vi "Meas.vi"(8 "error in (no error)":errorcluster, 10 "Variable":enum16{"Voltage", "Current"}(ring), 11 "Connection in":T1={"Baud"=9600, "Flow Ctl"=0, "COM port"="", "Parity"=0} {"Parity" items=["None", "Odd", "Even"]; "Flow Ctl" items=["None"]; "Baud" items=["4800"=4800, "9600"=9600, "19200"=19200, "38400"=38400]}) -> (0 "error out":errorcluster, 2 "Value":dbl, 3 "Connection out":T1={"Baud"=9600, "Flow Ctl"=0, "COM port"="", "Parity"=0} {"Parity" items=["None", "Odd", "Even"]; "Flow Ctl" items=["None"]; "Baud" items=["4800"=4800, "9600"=9600, "19200"=19200, "38400"=38400]})   [LabVIEW 2014, in "B&K Precision 9120 series.lvclass"]
uses:
  B&K Precision 9120 series.lvclass
  Serial_Config.ctl
  <vilib>/Utility/error.llb/DialogType.ctl
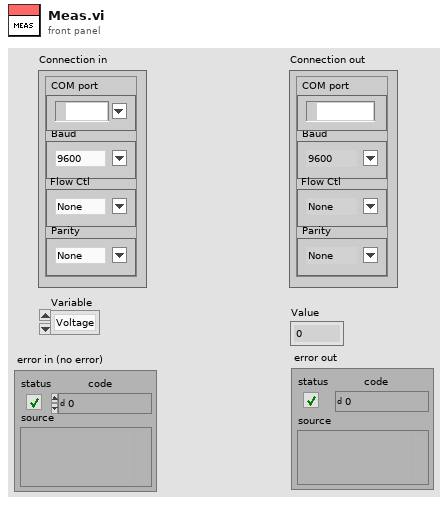
[diagram p1: front panel]
types:
  T1 = typedef "B&K Precision 9120 series.lvclass/Serial_Config.ctl" = cluster{"Baud":u32, "Flow Ctl":u16, "COM port":refnum<visa-resource-name>, "Parity":u16}
  T2 = typedef "DialogType.ctl" = u16
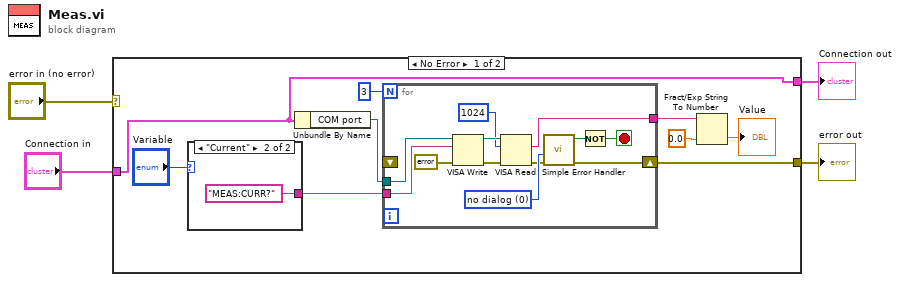
[diagram p0: block diagram]
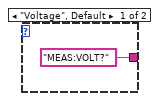
[diagram p2: hidden frame]
diagram:
  n1 = case shown="No Error" "error in (no error)" {
    selector: "error in (no error)" -> [_ w29]
    tunnel: [w6 w29] -> w4
    tunnel: "Connection in" -> [w5 w28]
    tunnel: [w5 w28] -> w1
    frame No Error {
      n2 = case shown="\"Current\"" "Variable" {
        tunnel: ["MEAS:VOLT?" ("write buffer") "MEAS:CURR?" ("write buffer")] -> w13
        frame "Voltage", Default {
        }
        frame "Current" {
        }
      }
      n3 = Unbundle By Name(w5) -> ("COM port"=w9:refnum<visa-resource-name>)
      n4 = for {
        N: 3 -> [_]
        tunnel: w13 -> [w24]
        tunnel: [w22] -> w11
        tunnel: w9 -> [w21]
        shift-right: [w15] -> w6
        shift-left: _ -> [_]
        stop <- w16 stop-if-true
        w19 = T2 0 items=["no dialog", "OK message", "continue or stop message", "OK message + warnings", "continue/stop + warnings"] ("type of dialog (OK msg:1)")
        n5 = VISA Write(VISA resource name=w21, write buffer=w24, error in (no error)=errorcluster {"status"=FALSE, "code"=0, "source"=""} ("error constant")) -> (VISA resource name out=w25:refnum<visa-resource-name>, error out=w20:errorcluster)  [unwired: 1 out]
        n6 = VISA Read(VISA resource name=w25, byte count=u32 1024, error in (no error)=w20) -> (read buffer=w22:string, error out=w18:errorcluster)  [unwired: 2 out]
        n7 = call <vilib>:"Simple Error Handler.vi"("type of dialog (OK msg:1)"=w19, "error in (no error)"=w18) -> ("error?"=w17:bool, "error out"=w15:errorcluster)  [unwired: 3 in, 3 out]
        n8 = Not(x=w17) -> (.not. x?=w16:bool)
      }
      n9 = Fract/Exp String To Number(string=w11, default (0 dbl)=0.0 ("default (0 I32)")) -> (number=→"Value":dbl)  [unwired: 2 in, 1 out]
    }
    frame Error {
    }
  }
  "error out" <- w4
  "Connection out" <- w1
